vi "Frame.Convert.Name.vi"(11 "VS Frame Name":string) -> (2 "ID":u16, 3 "Frame Name":string)   [LabVIEW 2019, in "Diagnostics Addon System Explorer.lvlib"]
uses:
  Diagnostics Addon System Explorer.lvlib
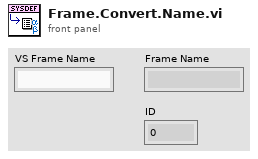
[diagram p1: front panel]
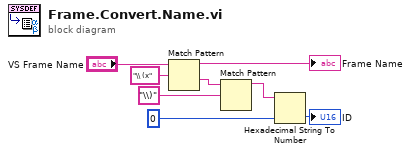
[diagram p0: block diagram]
diagram:
  n1 = Match Pattern(string="VS Frame Name", regular expression="\\ (x") -> (before substring=→"Frame Name":string, after substring=w3:string)  [unwired: 1 in, 2 out]
  n2 = Match Pattern(string=w3, regular expression="\\)") -> (before substring=w5:string)  [unwired: 1 in, 3 out]
  n3 = Hexadecimal String To Number(string=w5, default (0uL)=u16 0 ("default (0 U32)")) -> (number=→"ID":u16)  [unwired: 1 in, 1 out]
